vi "F-R.vi"(9 "Output Port":T2=3 items=["Port A", "Port B", "Port C", "All Ports"], 10 "Power (75)":i8=75, 11 "Foward/Reverse":bool) -> ()   [LabVIEW 2009]
uses:
  <vilib>/NXT/Subs/MotorOutput.ctl
  <vilib>/NXT/Subs/LVHSConnector.ctl
  <vilib>/NXT/Dual Mode Library/Motors/MotorReverse.vi
  <vilib>/NXT/Dual Mode Library/Motors/MotorOn.vi
panel:
  out "NXT 2":T1 caption="NXT"
  in  "NXT":T1
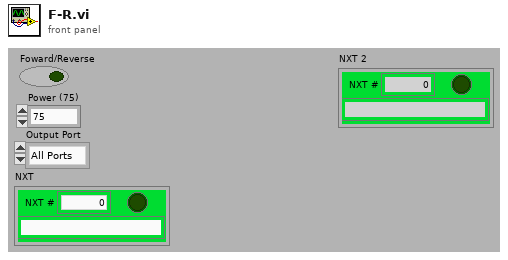
[diagram p1: front panel]
types:
  T1 = typedef "LVHSConnector.ctl" = cluster{"error":errorcluster, "address":string, "NXT #":i32, "Show Error":bool}
  T2 = typedef "MotorOutput.ctl" = u16
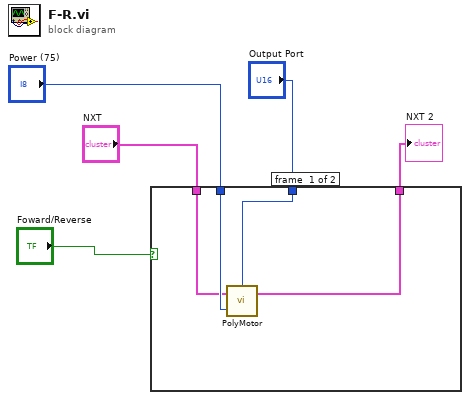
[diagram p0: block diagram]
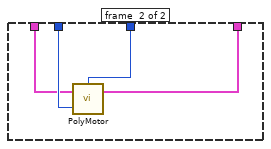
[diagram p2: hidden frame]
diagram:
  n1 = case shown="False" "Foward/Reverse" {
    tunnel: "Power (75)" -> [w9 w13]
    tunnel: "Output Port" -> [w8 w12]
    tunnel: "NXT" -> [w7 w11]
    tunnel: [w6 w10] -> w1
    frame #0 {
      n2 = call-poly <vilib>:"PolyMotor.vi"("Power (75)"=w9, "NXT"=w7, "Output Port"=w8) -> ("NXT"=w6:T1)  [unwired: 1 in]
    }
    frame #1 {
      n3 = call-poly <vilib>:"PolyMotor.vi"("Power (75)"=w13, "NXT"=w11, "Output Port"=w12) -> ("NXT"=w10:T1)  [unwired: 1 in]
    }
  }
  "NXT 2" <- w1
